vi "InstruGloble.vi"() -> ()   [LabVIEW 2012]
panel:
  out "Acqu.Count":u32
  out "Position":dbl[](array[numeric])
  in  "Save":bool
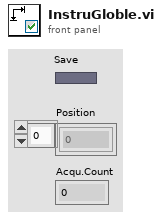
[diagram p1: front panel]
diagram:
